vi "Send Worker Status Update.vi"(8 "error in (no error)":errorcluster, 9 "Status":string, 10 "Operation":string, 11 "BuildWorker in":refnum<class "BuildWorker.lvclass">) -> (0 "error out":errorcluster, 3 "BuildWorker out":refnum<class "BuildWorker.lvclass">)   [LabVIEW 2017, in "BuildWorker.lvlib" / "BuildWorker.lvclass"]
uses:
  BuildWorker.lvclass
  Classes/Worker Status/Worker Status.lvclass
  Volumes/Data/Users/benji667/Git/BuildFarm/BuildWorker/Classes/Status/Status.lvclass
  BuildWorker.lvclass/BuildWorker.ctl
  WebSocket Server/Actors/WebSocket Client/WebSocket Client Messages/Send Message Msg/Send Message Msg.lvclass/Send Message Msg.ctl
  <vilib>/ActorFramework/Message Enqueuer/Message Enqueuer.lvclass/Message Enqueuer.ctl
  <vilib>/ActorFramework/Message Enqueuer/Enqueue.vi
  WebSocket Server/Actors/WebSocket Client/WebSocket Client Messages/Send Message Msg/Send Message Msg.lvclass
  Applications/National Instruments/LabVIEW 2017 64-bit/vi.lib/ActorFramework/Message/Message.lvclass
  <vilib>/ActorFramework/Message Priority Queue/Priority Enqueue.vi
  <vilib>/ActorFramework/Message Enqueuer/Message Enqueuer.lvclass
  Classes/Status/Status.lvclass
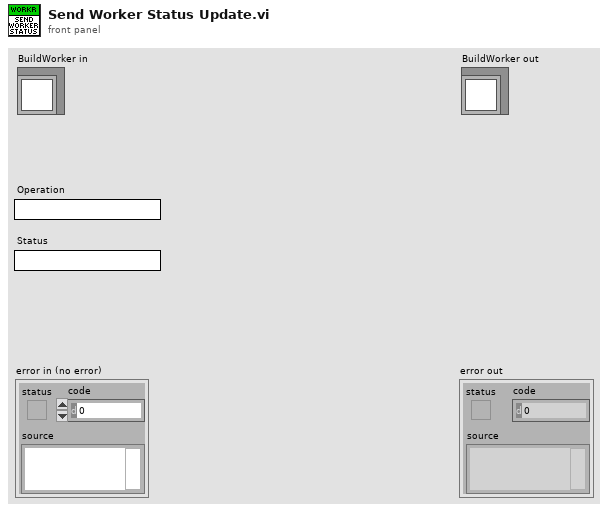
[diagram p1: front panel]
types:
  T1 = typedef "BuildWorker.lvlib/BuildWorker.lvclass/Status.ctl" = enum16{"Created", "Running", "Stopped", "On Error"}
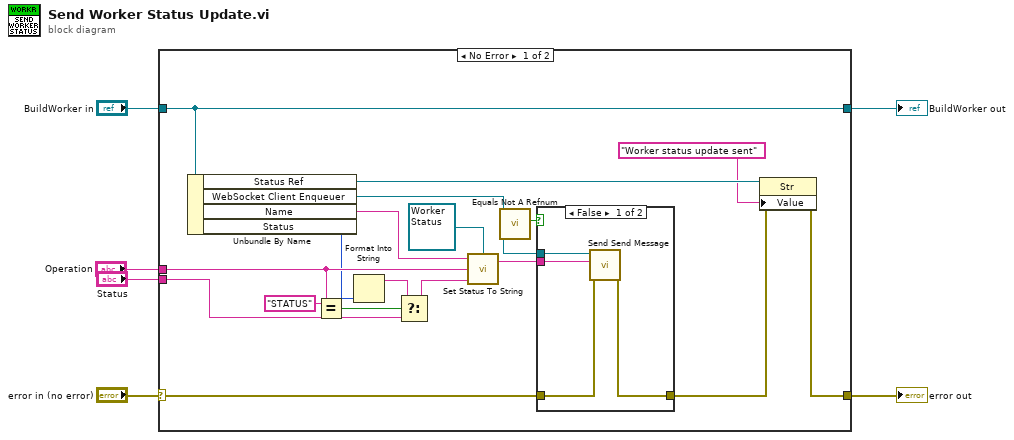
[diagram p0: block diagram]
diagram:
  n1 = case shown="No Error" "error in (no error)" {
    selector: "error in (no error)" -> [w23 w31]
    tunnel: [w19 w31] -> w5
    tunnel: [w24 w30] -> w3
    tunnel: "BuildWorker in" -> [w24 w30]
    tunnel: "Status" -> [w13 _]
    tunnel: "Operation" -> [w11 _]
    frame No Error {
      n2 = Unbundle By Name(w24) -> ("Status Ref"=w22:refnum<vi>, "WebSocket Client Enqueuer"=w18:refnum<class "Message Enqueuer.lvclass">, "Name"=w14:string, "Status"=w8:T1)
      n3 = Equal?(x="STATUS" ("y"), y=w11) -> (x = y?=w10:bool)
      n4 = Format Into String(w8) -> (resulting string=w7:string)  [unwired: 3 in, 1 out]
      n5 = Select(t=w7, s=w10, f=w13) -> (s? t:f=w12:string)
      n6 = call "Set Status To String.vi"("Status type"=refnum<class "Worker Status.lvclass"> refnum ("Worker Status.lvclass"), "Status"=w12, "Item Name"=w11, "Sender"=w14) -> ("data string"=w16:string)  [unwired: 1 in]
      n7 = call <vilib>:"Equals Not A Refnum.vi"("Message Enqueuer"=w18) -> ("Not a refnum?"=w17:bool)  [unwired: 10 in]
      n8 = case shown="False" w17 {
        tunnel: w18 -> [w28 _]
        tunnel: w23 -> [w27 w29]
        tunnel: [w26 w29] -> w20
        tunnel: w16 -> [w25 _]
        frame False {
          n9 = call "Send Send Message.vi"("error in (no error)"=w27, "Message"=w25, "Message Enqueuer in"=w28) -> ("error out"=w26:errorcluster)  [unwired: 7 in, 1 out]
        }
        frame True {
        }
      }
      n10 = property class="Str"(reference=w22, error in=w20, "Value"="Worker status update sent") -> (error out=w19:errorcluster)  [unwired: 1 out]
    }
    frame Error {
    }
  }
  "error out" <- w5
  "BuildWorker out" <- w3
